vi "SendTrig.vi"(8 "error in (no error)":errorcluster, 10 "Send vi Trig":bool, 11 "Instrument Handle":refnum<k15>) -> (0 "error out":errorcluster, 3 "Instrument Handle Out":refnum<k15>)   [LabVIEW 2020]
uses:
  <instrlib>/niFgen/niFgen.llb/niFgen_ctl Trigger SW - TrigName Values (Ring).ctl
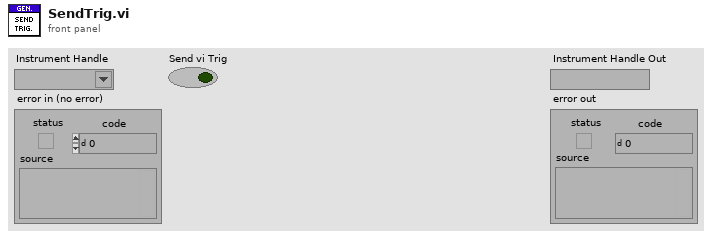
[diagram p1: front panel]
types:
  T1 = typedef "niFgen_ctl Trigger SW - TrigName Values (Ring).ctl" = i32
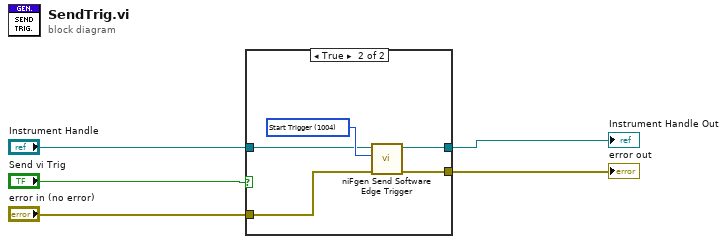
[diagram p0: block diagram]
diagram:
  n1 = case shown="True" "Send vi Trig" {
    tunnel: "Instrument Handle" -> [w7 w11]
    tunnel: "error in (no error)" -> [w6 w10]
    tunnel: [w7 w9] -> w3
    tunnel: [w6 w8] -> w2
    frame False {
    }
    frame True {
      w12 = T1 1004 items=["Start Trigger"=1004, "Script Trigger"=104] ("Trigger (Start Trigger)")
      n2 = call <instrlib>:"niFgen Send Software Edge Trigger.vi"("error in (no error)"=w10, "Trigger (Start Trigger)"=w12, "Instrument Handle"=w11) -> ("error out"=w8:errorcluster, "Instrument Handle Out"=w9:refnum<k15>)  [unwired: 7 in]
    }
  }
  "Instrument Handle Out" <- w3
  "error out" <- w2
